vi "Override Error.vi"(7 "Sender":refnum<class "Sender.lvclass">, 10 "Error":errorcluster, 11 "Base jettl in":refnum<class "Base jettl.lvclass">) -> (3 "Base jettl out":refnum<class "Base jettl.lvclass">)   [LabVIEW 2021, in "jettl.lvlib" / "Base jettl.lvclass"]
uses:
  Base jettl.lvclass
  Base jettl.lvclass/Base jettl.ctl
  State.ctl
  Sender/Sender/Sender.lvclass
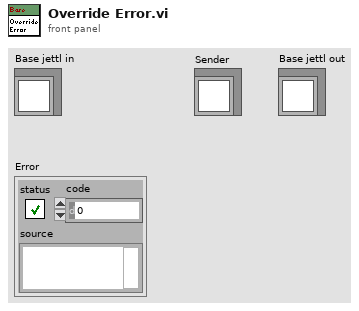
[diagram p1: front panel]
types:
  T1 = typedef "jettl.lvlib/Base jettl.lvclass/State.ctl" = enum16{"Nominal", "Teardown", "Error"}
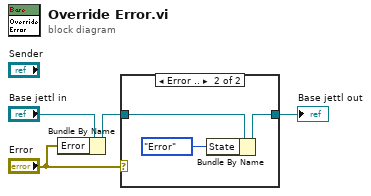
[diagram p0: block diagram]
diagram:
  n1 = Bundle By Name(cluster="Base jettl in", "Error"="Error") -> (w3:refnum<class "Base jettl.lvclass">)
  n2 = case shown="Error .." "Error" {
    tunnel: [w5 w7] -> w2
    tunnel: w3 -> [w5 w8]
    frame No Error {
    }
    frame Error {
      n3 = Bundle By Name(cluster=w8, "State"=State."Error") -> (w7:refnum<class "Base jettl.lvclass">)
    }
  }
  "Base jettl out" <- w2
